vi "监测块.vi"(10 "索引":i32, 11 "数组":u16[](array[numeric])) -> (1 "string":string, 2 "数值":sgl, 3 "time stamp":timestamp)   [LabVIEW 2016, in "斯坦道总磷总氮V2.lvlib"]
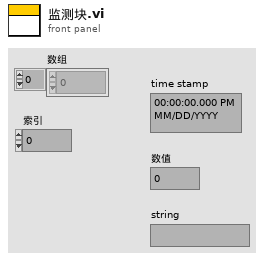
[diagram p1: front panel]
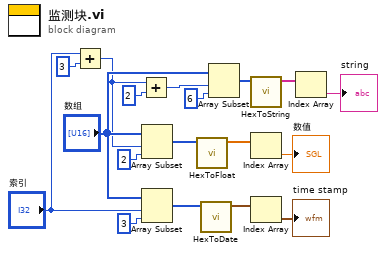
[diagram p0: block diagram]
diagram:
  n1 = Add(x="索引", y=3) -> (x+y=w3:i32)
  n2 = Add(x=w3, y=2) -> (x+y=w1:i32)
  n3 = Array Subset(array="数组", index=w3, length=2 ("长度")) -> (w12:u16[])
  n4 = Array Subset(array="数组", index="索引", length=3 ("长度")) -> (w7:u16[])
  n5 = call "HexToFloat.vi"("数组"=w12) -> ("FLOAT"=w13:sgl[])  [unwired: 10 in]
  n6 = call "HexToDate.vi"("数组"=w7) -> ("DATE"=w8:timestamp[])  [unwired: 10 in]
  n7 = Array Subset(array="数组", index=w1, length=6 ("长度")) -> (w16:u16[])
  n8 = call "HexToString.vi"("数组"=w16) -> ("STRING"=w17:string[])  [unwired: 10 in]
  n9 = Index Array(array=w13) -> (element=→"数值":sgl)  [unwired: 1 in]
  n10 = Index Array(array=w8) -> (element=→"time stamp":timestamp)  [unwired: 1 in]
  n11 = Index Array(array=w17) -> (element=→"string":string)  [unwired: 1 in]
